vi "4-6（3）.vi"() -> ()   [LabVIEW 2017]
panel:
  in  "停止":bool
  out "和":dbl
  in  "加数 2":dbl
  in  "加数1":dbl
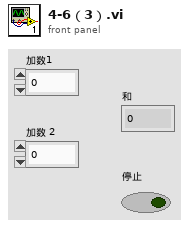
[diagram p1: front panel]
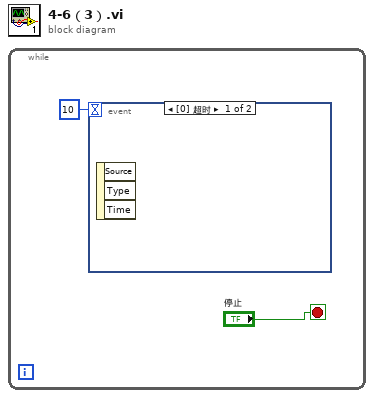
[diagram p0: block diagram]
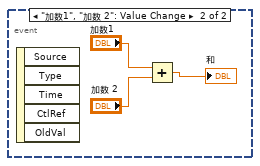
[diagram p2: hidden frame]
diagram:
  n1 = while {
    stop <- "停止" stop-if-true
    n2 = event shown="[0] 超时" {
      selector: _ -> [_ _]
      dyn-events: _ -> [_ _]
      timeout: 10 -> [_ _]
      event Timeout {
        n3 = event-data() -> ()  [unwired: 1 in, 3 out]
      }
      event "加数1", "加数 2": Value Change {
        n4 = event-data() -> ()  [unwired: 1 in, 5 out]
        n5 = Add(x="加数1", y="加数 2") -> (x+y=→"和":dbl)
      }
    }
  }
